vi "ZCAN_Filter.vi"(7 "error in (no error)":errorcluster caption="错误输入（无错误）", 9 "can_index":u32, 10 "device_handle":u32) -> (0 "error out":errorcluster caption="错误输出")   [LabVIEW 2021, in "zlgcan.lvlib"]
doc: "设置滤波，最多设置50条\n在SubVI内部设置，可根据项目实际需求修改\n在Init 初始化之后， Start 之前使用\n\n适用型号：USBCANFD-100U、USBCANFD-200U、USBCANFD-MINI、\nPCI-5010-U、PCI-5020-U、USBCAN-E-U、USBCAN-2E-U、CANalyst-II+、\nUSBCAN-4E-U"
uses:
  zlgcan.lvlib
panel:
  # "在后面板添加滤波表格"
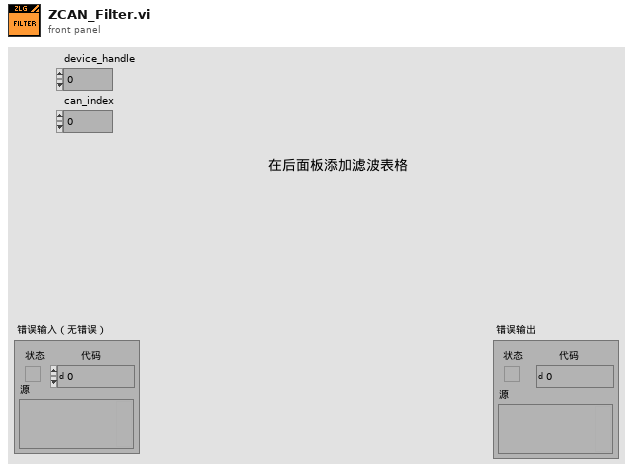
[diagram p1: front panel]
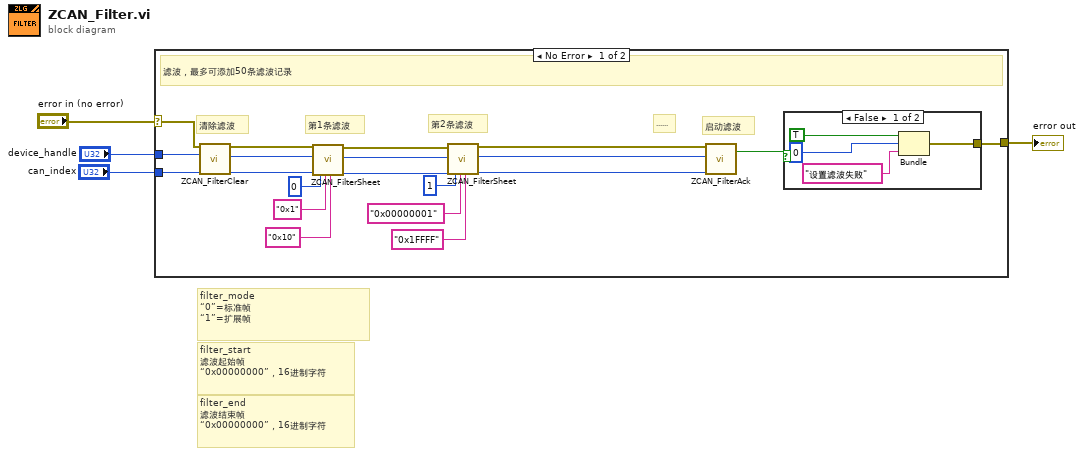
[diagram p0: block diagram]
diagram:
  # "filter_end\n滤波结束帧\n“0x00000000”，16进制字符"
  # "filter_start   \n滤波起始帧 \n“0x00000000”，16进制字符"
  # "filter_mode\n“0”=标准帧\n“1”=扩展帧"
  n1 = case shown="No Error" "error in (no error)" {
    selector: "error in (no error)" -> [w23 w29]
    tunnel: [w24 w29] -> w3
    tunnel: "device_handle" -> [w22 _]
    tunnel: "can_index" -> [w21 _]
    frame No Error {
      # "......"
      # "启动滤波"
      # "第2条滤波"
      # "清除滤波"
      # "第1条滤波"
      # "滤波，最多可添加50条滤波记录"
      n2 = call "ZCAN_FilterClear.vi"("error in (no error)"=w23, "can_index_handle"=w22, "can_index"=w21) -> ("error out"=w14:errorcluster, "can_index_handle(out)"=w19:u32, "can_index(out)"=w18:u32)  [unwired: 14 in]
      n3 = call "ZCAN_FilterSheet.vi"("error in (no error)"=w14, "can_index_handle"=w19, "can_index"=w18, "filter_mode"=u32 0, "filter_start"="0x1", "filter_end"="0x10") -> ("error out"=w17:errorcluster, "can_index_handle（out）"=w16:u32, "can_index (out)"=w15:u32)  [unwired: 11 in]
      n4 = call "ZCAN_FilterSheet.vi"("error in (no error)"=w17, "can_index_handle"=w16, "can_index"=w15, "filter_mode"=u32 1, "filter_start"="0x00000001", "filter_end"="0x1FFFF") -> ("error out"=w7:errorcluster, "can_index_handle（out）"=w6:u32, "can_index (out)"=w5:u32)  [unwired: 11 in]
      n5 = call "ZCAN_FilterAck.vi"("error in (no error)"=w7, "can_index_handle"=w6, "can_index"=w5) -> ("启动滤波成功？"=w20:bool)  [unwired: 13 in, 3 out]
      n6 = case shown="False" w20 {
        tunnel: [w25 _] -> w24
        frame False {
          n7 = Bundle("status"=TRUE, "code"=0, "消息"="设置滤波失败") -> (w25:cluster{"status":bool, "code":i32, "消息":string})  [unwired: 1 in]
        }
        frame True {
        }
      }
    }
    frame Error {
    }
  }
  "error out" <- w3
